vi "Create update clock (AO).vi"(8 "error in":errorcluster, 11 "RUS settings":T1={"NI-DAQ lockin settings"={"Samples per sine wave"=0, "Sine waves per freq step"=0, "Output Representation"=enum."Real/Imaginary", "Low-pass filter"=enum."Butterworth", "Ranges and couplings "=[]}, "Fast swep settings"={"Update rate (Hz)"=250.0, "Start F, Hz"=200000.0, "Stop F"=1700000.0, "Number of points"=30000, "Amplitude"=2.1, "Init&amplitude"=TRUE, "IF"=1000.0, "Time constant"=0.1}, "Pre-sweep delay, s"=0.0, "Lockin mode"=enum."NI-DAQ", "SR Lockin"="GPIB0::10::INSTR", "DAQmx Device"="Dev3", "Clock Multiplier"=64, "Fast Sweep Data Out"={"DO clock task"="", "DO task"="", "Update clock task"="", "DAQ lockin task"="", "Pre-sweep counter task"=""}, "Lockin Range, V"=0.0, "F Array"=[], "Freq. update clock terminal"="", "DO Clock Rate (Hz)"=5000000.0, "ADC clock terminal"="/PFI4", "Pre-sweep counter terminal"="/PFI4", "Samples per read"=10, "DO clock terminal"="", "Pre-sweep points"=0, "F points per write"=0, "Total sweep time, s"=1000.0, "Initial SYNTH phase"=0.0, "Record IF"=FALSE, "Save data settings"={"Save data"=TRUE, "Data Root Path"=path "", "File Prefix"="", "File Format"=enum."ASCII", "Save column names"=TRUE, "File Comments"="<Description of the current file>", "User/Prj"="<User Name/Project Description>"}, "Data file path"=path "", "New data user event"=refnum, "Stop user event"=refnum, "Number of channels"=1, "Auto-phase"=FALSE} {"Lockin Range, V" format="%#_6e"; "Fast swep settings"."IF" format="%#_6p"; "Fast swep settings"."Amplitude" min=0.0 max=2.5; "Fast swep settings"."Number of points" format="%.0p"; "Fast swep settings"."Stop F" format="%#_6p"; "Fast swep settings"."Start F, Hz" format="%#_6p"; "Fast swep settings"."Update rate (Hz)" format="%0.2f"; "NI-DAQ lockin settings"."Ranges and couplings"."Coupling" items=["default"=-1, "RSE"=10083, "NRSE"=10078, "Differential"=10106, "Pseudodifferential"=12529]}) -> (0 "error out":errorcluster, 3 "RUS settings out":T1={"NI-DAQ lockin settings"={"Samples per sine wave"=0, "Sine waves per freq step"=0, "Output Representation"=enum."Real/Imaginary", "Low-pass filter"=enum."Butterworth", "Ranges and couplings "=[]}, "Fast swep settings"={"Update rate (Hz)"=250.0, "Start F, Hz"=200000.0, "Stop F"=1700000.0, "Number of points"=30000, "Amplitude"=2.1, "Init&amplitude"=TRUE, "IF"=1000.0, "Time constant"=0.1}, "Pre-sweep delay, s"=0.0, "Lockin mode"=enum."NI-DAQ", "SR Lockin"="GPIB0::10::INSTR", "DAQmx Device"="Dev3", "Clock Multiplier"=64, "Fast Sweep Data Out"={"DO clock task"="", "DO task"="", "Update clock task"="", "DAQ lockin task"="", "Pre-sweep counter task"=""}, "Lockin Range, V"=0.0, "F Array"=[], "Freq. update clock terminal"="", "DO Clock Rate (Hz)"=5000000.0, "ADC clock terminal"="/PFI4", "Pre-sweep counter terminal"="/PFI4", "Samples per read"=10, "DO clock terminal"="", "Pre-sweep points"=0, "F points per write"=0, "Total sweep time, s"=1000.0, "Initial SYNTH phase"=0.0, "Record IF"=FALSE, "Save data settings"={"Save data"=TRUE, "Data Root Path"=path "", "File Prefix"="", "File Format"=enum."ASCII", "Save column names"=TRUE, "File Comments"="<Description of the current file>", "User/Prj"="<User Name/Project Description>"}, "Data file path"=path "", "New data user event"=refnum, "Stop user event"=refnum, "Number of channels"=1, "Auto-phase"=FALSE} {"Lockin Range, V" format="%#_6e"; "Fast swep settings"."IF" format="%#_6p"; "Fast swep settings"."Amplitude" min=0.0 max=2.5; "Fast swep settings"."Number of points" format="%.0p"; "Fast swep settings"."Stop F" format="%#_6p"; "Fast swep settings"."Start F, Hz" format="%#_6p"; "Fast swep settings"."Update rate (Hz)" format="%0.2f"; "NI-DAQ lockin settings"."Ranges and couplings"."Coupling" items=["default"=-1, "RSE"=10083, "NRSE"=10078, "Differential"=10106, "Pseudodifferential"=12529]})   [LabVIEW 2015]
uses:
  RUS/Controls/RUS settings.ctl
  RUS/Controls/RUS NI-DAQ Lockin Settings.ctl
  RUS/Controls/Sweep settings.ctl
  NHMFL_Core/Libraries/File/Controls/Save data settings.ctl
  NHMFL_Core/Libraries/File/Controls/File formats.ctl
  <vilib>/DAQmx/write.llb/DAQmx Write (Analog 1D DBL 1Chan NSamp).vi
  <vilib>/DAQmx/create/channels.llb/DAQmx Create Channel (AO-Voltage-Basic).vi
  <vilib>/DAQmx/configure/timing.llb/DAQmx Timing (Sample Clock).vi
  <vilib>/DAQmx/miscellaneous.llb/DAQmx Fill In Error Info.vi
  <vilib>/DAQmx/create/channels.llb/DAQmx Create Channel (CO-Pulse Generation-Ticks).vi
  <vilib>/DAQmx/configure/trigger.llb/DAQmx Start Trigger (Digital Edge).vi
  <vilib>/DAQmx/configure/timing.llb/DAQmx Timing (Implicit).vi
  <resource>/objmgr/daqmx.rc
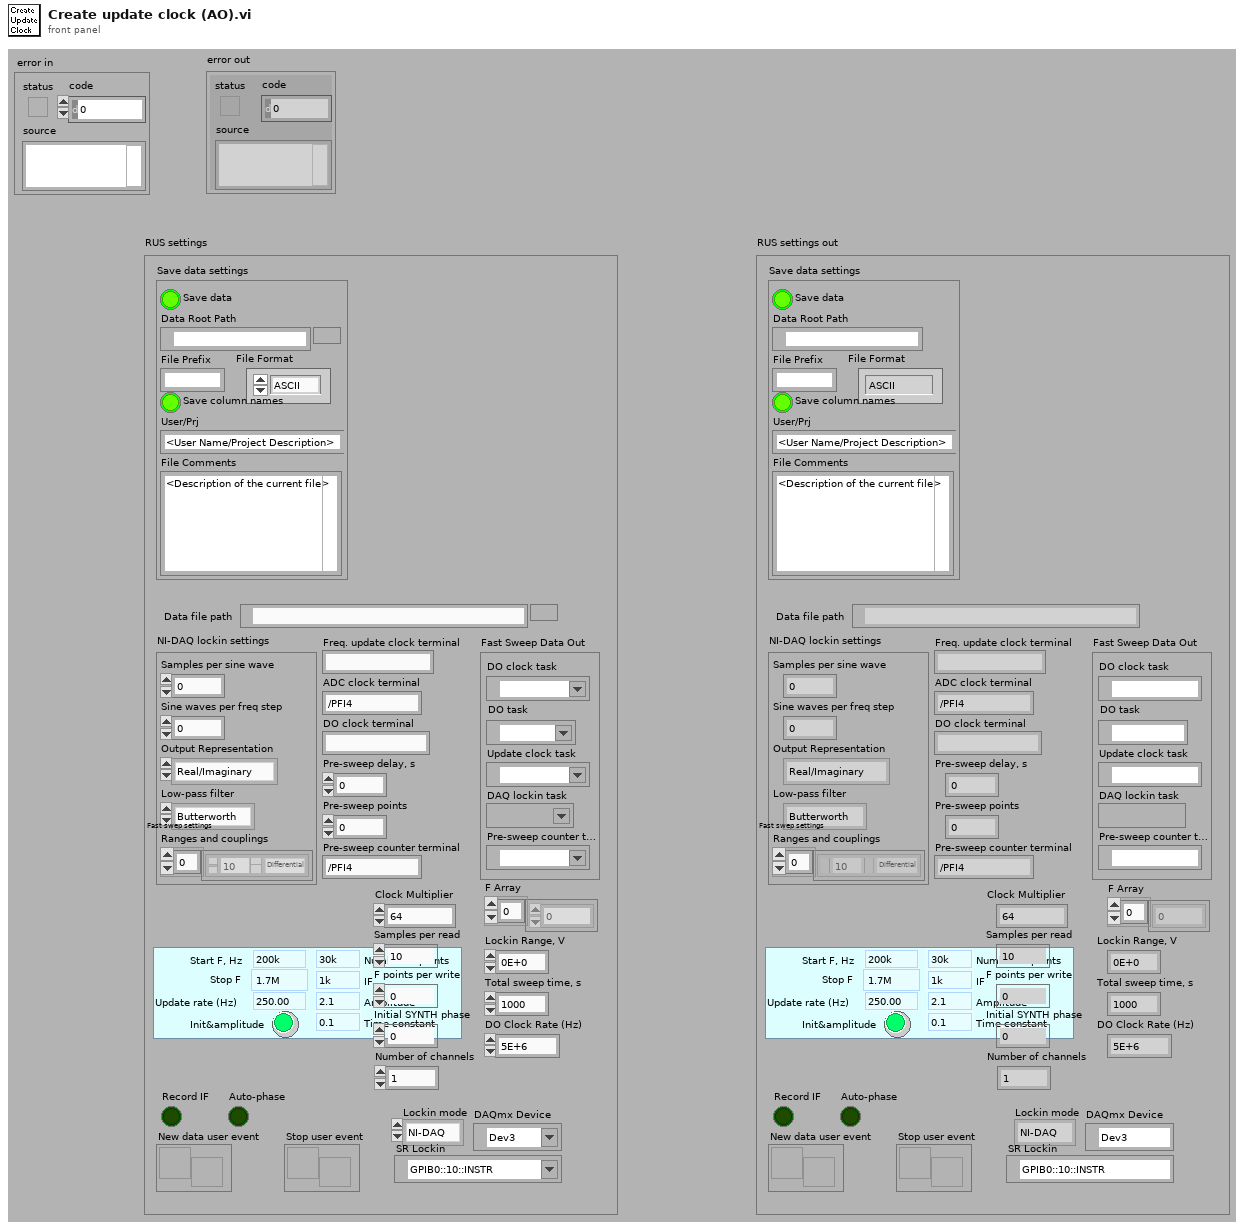
[diagram p1: front panel]
types:
  T1 = typedef "RUS settings.ctl" = cluster{"NI-DAQ lockin settings":T2, "Fast swep settings":T3, "Pre-sweep delay, s":dbl, "Lockin mode":enum16{"SRS", "NI-DAQ"}, "SR Lockin":refnum<visa-resource-name>, "DAQmx Device":tag, "Clock Multiplier":i32, "Fast Sweep Data Out":cluster{"DO clock task":refnum<k21>, "DO task":refnum<k21>, "Update clock task":refnum<k21>, "DAQ lockin task":refnum<k21>, "Pre-sweep counter task":refnum<k21>}, "Lockin Range, V":sgl, "F Array":dbl[], "Freq. update clock terminal":string, "DO Clock Rate (Hz)":dbl, "ADC clock terminal":string, "Pre-sweep counter terminal":string, "Samples per read":i32, "DO clock terminal":string, "Pre-sweep points":i32, "F points per write":i32, "Total sweep time, s":dbl, "Initial SYNTH phase":dbl, "Record IF":bool, "Save data settings":T4, "Data file path":path, "New data user event":refnum<user-event>, "Stop user event":refnum<user-event>, "Number of channels":i32, "Auto-phase":bool}
  T2 = typedef "RUS NI-DAQ Lockin Settings.ctl" = cluster{"Samples per sine wave":i32, "Sine waves per freq step":i32, "Output Representation":enum16{"Real/Imaginary", "Polar"}, "Low-pass filter":enum16{"No filtering", "Butterworth", "Bessel"}, "Ranges and couplings ":cluster{"Range":dbl, "Coupling":i32}[]}
  T3 = typedef "Sweep settings.ctl" = cluster{"Update rate (Hz)":dbl, "Start F, Hz":dbl, "Stop F":dbl, "Number of points":i32, "Amplitude":dbl, "Init&amplitude":bool, "IF":dbl, "Time constant":dbl}
  T4 = typedef "Save data settings.ctl" = cluster{"Save data":bool, "Data Root Path":path, "File Prefix":string, "File Format":T5, "Save column names":bool, "File Comments":string, "User/Prj":string}
  T5 = typedef "File formats.ctl" = enum16{"TDMS", "ASCII", "BINARY"}
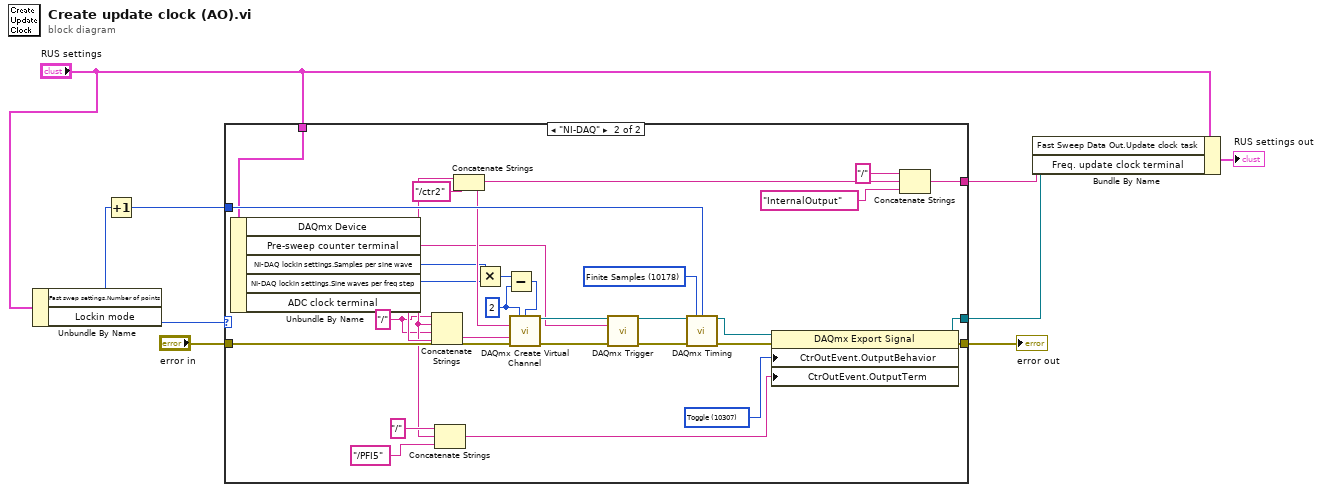
[diagram p0: block diagram]
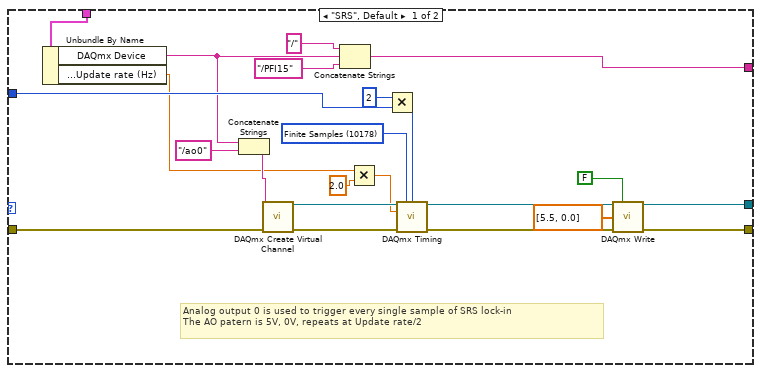
[diagram p2: hidden frame]
diagram:
  n1 = Unbundle By Name("RUS settings") -> ("Fast swep settings.Number of points"=w1:i32, "Lockin mode"=w6:enum16{"SRS", "NI-DAQ"})
  n2 = Increment(x=w1) -> (x+1=w7:i32)
  n3 = case shown="\"NI-DAQ\"" w6 {
    tunnel: [w25 w54] -> w9
    tunnel: [w24 w52] -> w4
    tunnel: [w19 w57] -> w2
    tunnel: "error in" -> [w14 w62]
    tunnel: w7 -> [w13 w60]
    tunnel: "RUS settings" -> [w12 w42]
    frame "SRS", Default {
      w29 = 10178 items=["Finite Samples"=10178, "Continuous Samples"=10123, "Hardware Timed Single Point"=12522] ("sample mode")
      # "Analog output 0 is used to trigger every single sample of SRS lock-in \nThe AO patern is 5V, 0V, repeats at Update rate/2"
      n4 = Unbundle By Name(w12) -> ("DAQmx Device"=w11:tag, "Fast swep settings.Update rate (Hz)"=w10:dbl)
      n5 = Concatenate Strings(w11, "/ao0") -> (w21:string)
      n6 = call-poly <vilib>:"DAQmx Create Virtual Channel.vi"("physical channels"=w21, "error in"=w14) -> ("task out"=w32:refnum<k21>, "error out"=w30:errorcluster)  [unwired: 7 in, 5 out]
      n7 = Concatenate Strings("/", w11, "/PFI15") -> (w19:string)
      n8 = Multiply(x=w10, y=2.0) -> (x*y=w16:dbl)
      n9 = Multiply(x=2 ("y"), y=w13) -> (x*y=w18:i32)
      n10 = call-poly <vilib>:"DAQmx Timing.vi"("task/channels in"=w32, "sample mode"=w29, "samples per channel"=w18, "rate"=w16, "error in"=w30) -> ("task out"=w31:refnum<k21>, "error out"=w28:errorcluster)  [unwired: 2 in, 7 out]
      n11 = call-poly <vilib>:"DAQmx Write.vi"("task/channels in"=w31, "auto start"=FALSE, "data"=dbl[] [5.5, 0.0], "error in"=w28) -> ("task out"=w24:refnum<k21>, "error out"=w25:errorcluster)  [unwired: 10 out]
    }
    frame "NI-DAQ" {
      w33 = "/"
      w48 = u32 2 ("high ticks")
      w53 = 10307 items=["Pulse"=10265, "Toggle"=10307] ("CtrOutEvent.OutputBehavior")
      w61 = 10178 items=["Finite Samples"=10178, "Continuous Samples"=10123, "Hardware Timed Single Point"=12522] ("sample mode")
      n12 = Unbundle By Name(w42) -> ("DAQmx Device"=w40:tag, "Pre-sweep counter terminal"=w35:string, "NI-DAQ lockin settings.Samples per sine wave"=w51:i32, "NI-DAQ lockin settings.Sine waves per freq step"=w50:i32, "ADC clock terminal"=w41:string)
      n13 = Concatenate Strings(w33, w40, w33, w41) -> (w43:string)
      n14 = Concatenate Strings("/", w40, "/PFI5" ("string")) -> (w44:string)
      n15 = Concatenate Strings(w40, "/ctr2") -> (w58:string)
      n16 = Multiply(x=w51, y=w50) -> (x*y=w49:i32)
      n17 = Subtract(x=w49, y=w48) -> (x-y=w47:u32)
      n18 = call-poly <vilib>:"DAQmx Create Virtual Channel.vi"("high ticks"=w48, "low ticks"=w47, "counter"=w58, "source of ticks"=w43, "error in"=w62) -> ("task out"=w38:refnum<k21>, "error out"=w39:errorcluster)  [unwired: 4 in, 5 out]
      n19 = call-poly <vilib>:"DAQmx Trigger.vi"("task/channels in"=w38, "source"=w35, "error in"=w39) -> ("task out"=w36:refnum<k21>, "error out"=w37:errorcluster)  [unwired: 11 in]
      n20 = call-poly <vilib>:"DAQmx Timing.vi"("task/channels in"=w36, "sample mode"=w61, "samples per channel"=w60, "error in"=w37) -> ("task out"=w34:refnum<k21>, "error out"=w55:errorcluster)  [unwired: 10 out]
      n21 = property class="DAQmx Export Signal"(reference=w34, error in=w55, "CtrOutEvent.OutputBehavior"=w53, "CtrOutEvent.OutputTerm"=w44) -> (reference out=w52:refnum<k21>, error out=w54:errorcluster)
      n22 = Concatenate Strings("/", w58, "InternalOutput" ("string")) -> (w57:string)
    }
  }
  "error out" <- w9
  n23 = Bundle By Name(cluster="RUS settings", "Fast Sweep Data Out.Update clock task"=w4, "Freq. update clock terminal"=w2) -> (→"RUS settings out":T1)
